vi "Shutdown.vi"(8 "error in (no error)":errorcluster, 11 "TCP Process in":refnum<class "TCP Process.lvclass">) -> (0 "error out":errorcluster)   [LabVIEW 2019, in "TimingDRV Engine.lvlib" / "TCP Process.lvclass"]
uses:
  TCP Process.lvclass
  TCP Process.lvclass/TCP Process.ctl
  Parent Classes/Process/Process.lvclass
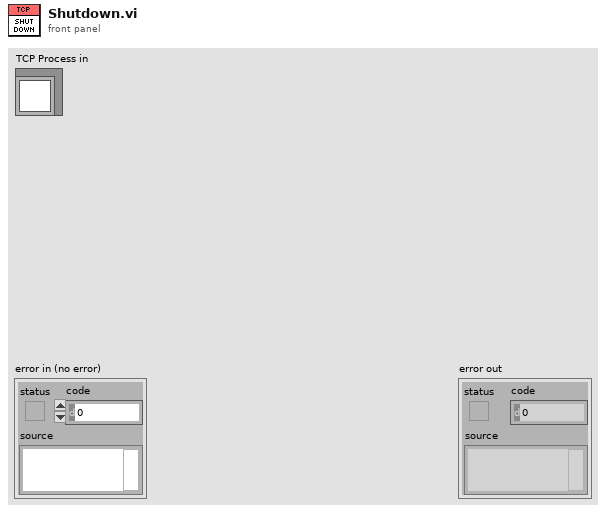
[diagram p1: front panel]
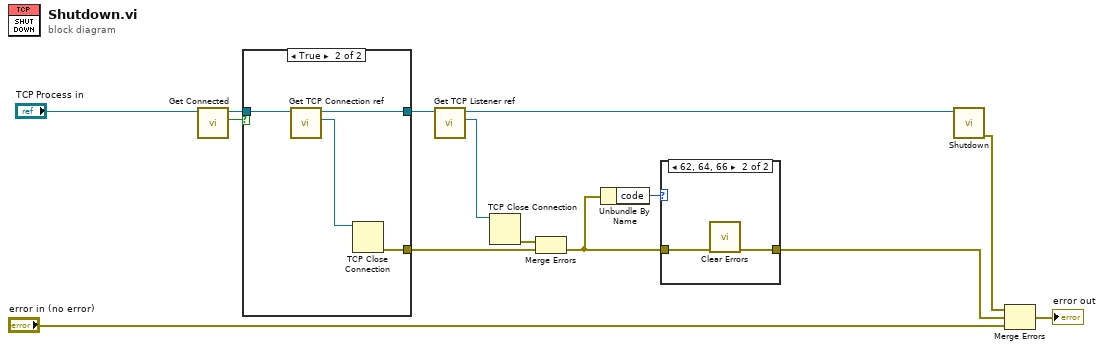
[diagram p0: block diagram]
diagram:
  n1 = call "Get Connected.vi"("TCP Process in"="TCP Process in") -> ("Connected"=w14:bool, "TCP Process out"=w13:refnum<class "TCP Process.lvclass">)  [unwired: 9 in]
  n2 = case shown="True" w14 {
    tunnel: w13 -> [w15 w19]
    tunnel: [w15 w17] -> w12
    tunnel: [_ w16] -> w10
    frame False {
    }
    frame True {
      n3 = call "Get TCP Connection ref.vi"("TCP Process in"=w19) -> ("TCP Connection ref"=w18:refnum<k5>, "TCP Process out"=w17:refnum<class "TCP Process.lvclass">)  [unwired: 9 in]
      n4 = TCP Close Connection(connection ID=w18) -> (error out=w16:errorcluster)  [unwired: 2 in, 1 out]
    }
  }
  n5 = call "Get TCP Listener ref.vi"("TCP Process in"=w12) -> ("Connection ref"=w11:refnum<k5>, "TCP Process out"=w5:refnum<class "TCP Process.lvclass">)  [unwired: 9 in]
  n6 = TCP Close Connection(connection ID=w11) -> (error out=w9:errorcluster)  [unwired: 2 in, 1 out]
  n7 = Merge Errors(w9, w10) -> (w8:errorcluster)
  n8 = Unbundle By Name(w8) -> ("code"=w7:i32)
  n9 = case shown="62, 64, 66" w7 {
    tunnel: w8 -> [w20 w22]
    tunnel: [w20 w21] -> w3
    frame Default {
    }
    frame 62, 64, 66 {
      n10 = call <vilib>:"Clear Errors.vi"("error in (no error)"=w22) -> ("error out"=w21:errorcluster)  [unwired: 5 in, 1 out]
    }
  }
  n11 = call-parent "Shutdown.vi"("Process in"=w5) -> ("error out"=w4:errorcluster)  [unwired: 10 in]
  n12 = Merge Errors(w4, w3, "error in (no error)") -> (→"error out":errorcluster)
